vi "pcap-close.vi"(0 "Opened":bool) -> ()   [LabVIEW 2017]
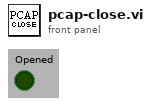
[diagram p1: front panel]
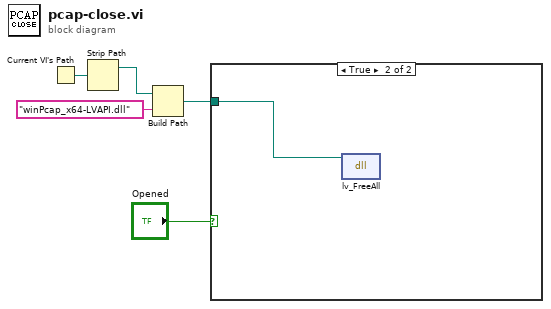
[diagram p0: block diagram]
diagram:
  n1 = Current VI's Path() -> (path=w4:path)
  n2 = Strip Path(path=w4) -> (stripped path=w3:path)  [unwired: 1 out]
  n3 = Build Path(base path=w3, name or relative path="winPcap_x64-LVAPI.dll") -> (appended path=w1:path)
  n4 = case shown="True" "Opened" {
    tunnel: w1 -> [_ w6]
    frame False {
    }
    frame True {
      n5 = dll-call lib="C:/Users/ucbtspu.AD/OneDrive - University College London/Local SCC/SilverLab-Microscope x64/Ethernet/winPcap_x64-LVAPI.dll" fn="lv_FreeAll"(path in=w6) -> ()  [unwired: 3 in, 2 out]
    }
  }
